vi "ErrortoString.vi"(8 "error in (no error)":errorcluster) -> (3 "String":string)   [LabVIEW 2017, in "Error Handler_JKI.lvlib"]
uses:
  APIs/Error Handler_JKI.lvlib
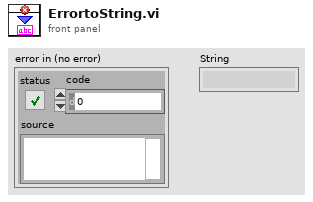
[diagram p1: front panel]
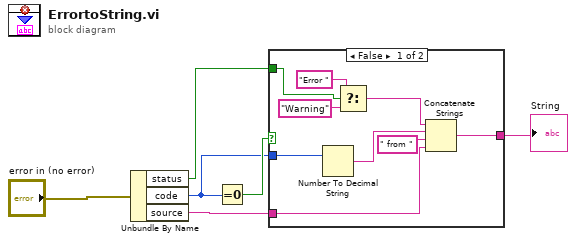
[diagram p0: block diagram]
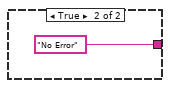
[diagram p2: hidden frame]
diagram:
  n1 = Unbundle By Name("error in (no error)") -> ("status"=w4:bool, "code"=w2:i32, "source"=w1:string)
  n2 = Equal To 0?(x=w2) -> (x = 0?=w3:bool)
  n3 = case shown="False" w3 {
    tunnel: [w10 "No Error"] -> w5
    tunnel: w1 -> [w8 _]
    tunnel: w2 -> [w9 _]
    tunnel: w4 -> [w7 _]
    frame False {
      n4 = Number To Decimal String(number=w9) -> (decimal integer string=w12:string)  [unwired: 1 out]
      n5 = Select(t="Error ", s=w7, f="Warning") -> (s? t:f=w13:string)
      n6 = Concatenate Strings(w13, w12, " from " ("string"), w8) -> (w10:string)
    }
    frame True {
    }
  }
  "String" <- w5
